vi "IC_ActiveBuffer_to_Picture.vi"(0 "ICImagingControl In":refnum<k7>, 1 "Error In (no error)":errorcluster) -> (2 "ICImagingControl Out":refnum<k7>, 3 "Picture Out":picture, 4 "SampleStartTime":dbl, 5 "Error Out":errorcluster)   [LabVIEW 2015]
uses:
  <vilib>/picture/picture.llb/Draw 8-Bit Pixmap.vi
  <vilib>/picture/picture.llb/Draw True-Color Pixmap.vi
  IC LabVIEW Extension 2.dll
  IC LabVIEW Extension 2.dll 
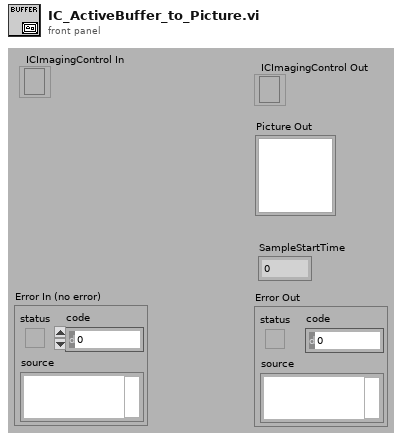
[diagram p1: front panel]
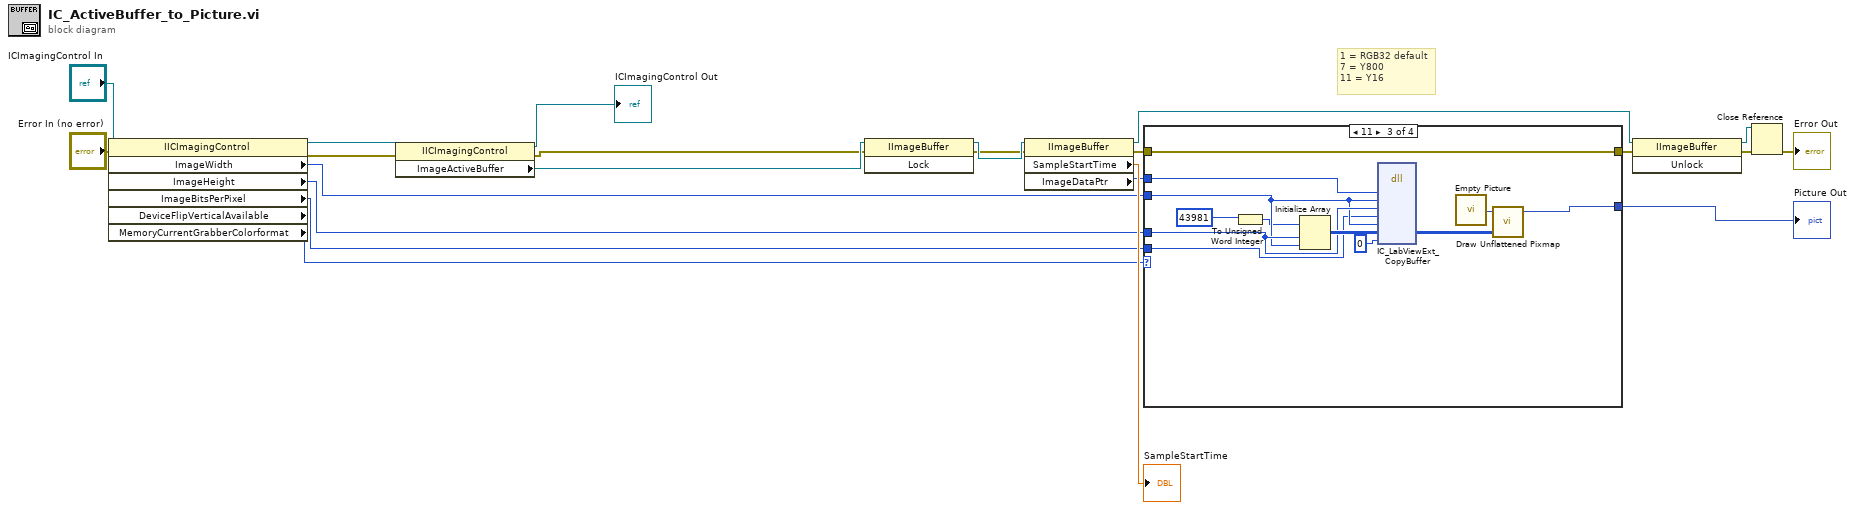
[diagram p0: block diagram]
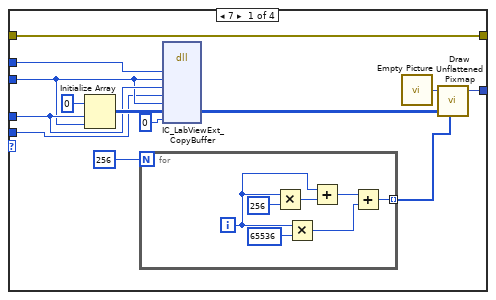
[diagram p2: hidden frame]
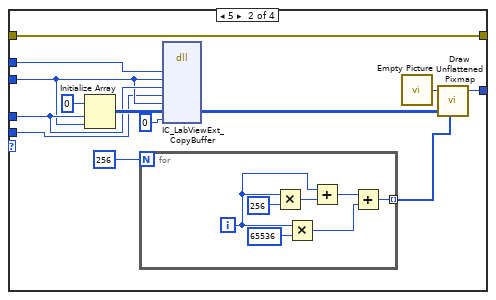
[diagram p3: hidden frame]
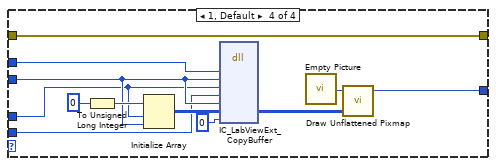
[diagram p4: hidden frame]
diagram:
  # "1 = RGB32 default\n7 = Y800\n11 = Y16"
  n1 = property class="IICImagingControl" props=["ImageWidth", "ImageHeight", "ImageBitsPerPixel", "DeviceFlipVerticalAvailable", "MemoryCurrentGrabberColorformat"](reference="ICImagingControl In", error in="Error In (no error)") -> (reference out=w6:refnum<k7>, error out=w4:errorcluster, "ImageWidth"=w12:i32, "ImageHeight"=w13:i32, "ImageBitsPerPixel"=w11:i32, "MemoryCurrentGrabberColorformat"=w14:i32)  [unwired: 1 out]
  n2 = property class="IICImagingControl"(reference=w6, error in=w4) -> (reference out=→"ICImagingControl Out":refnum<k7>, error out=w2:errorcluster, "ImageActiveBuffer"=w3:refnum<k7>)
  n3 = invoke class="IImageBuffer" method="Lock"(reference=w3, error in=w2) -> (reference out=w15:refnum<k7>, error out=w1:errorcluster)  [unwired: 1 in, 1 out]
  n4 = property class="IImageBuffer"(reference=w15, error in=w1) -> (reference out=w20:refnum<k7>, error out=w8:errorcluster, "SampleStartTime"=→"SampleStartTime":dbl, "ImageDataPtr"=w10:i32)
  n5 = case shown="11" w14 {
    tunnel: w13 -> [w28 w48 w70 w79]
    tunnel: w12 -> [w27 w47 w69 w80]
    tunnel: w11 -> [w26 w46 w68 w78]
    tunnel: w10 -> [w25 w45 w67 w77]
    tunnel: [w24 w44 w66 w76] -> w9
    tunnel: w8 -> [w23 w43 w65 w75]
    tunnel: [w23 w43 w65 w75] -> w7
    frame 7 {
      n6 = Initialize Array(u8 0, w28, w27) -> (w31:u8[][])
      n7 = for {
        N: 256 -> [_]
        tunnel: [w36] -> w32 mode=indexing
        i -> [w37]
        n8 = Multiply(x=w37, y=256) -> (x*y=w40:i32)
        n9 = Multiply(x=w37, y=65536) -> (x*y=w42:i32)
        n10 = Add(x=w37, y=w40) -> (x+y=w38:i32)
        n11 = Add(x=w38, y=w42) -> (x+y=w36:i32)
      }
      n12 = dll-call lib="IC LabVIEW Extension 2.dll " fn="IC_LabViewExt_CopyBuffer"("data"=w25, "width"=w27, "height"=w28, "bpp"=w26, "imaq_width"=w27, "imaq_ptr"=w31, "bFlip"=0) -> ("imaq_ptr"=w29:u8[][])  [unwired: 10 in, 2 out]
      n13 = call "Empty Picture"() -> ("empty picture"=w35:picture)
      n14 = call-poly <vilib>:"Draw Unflattened Pixmap.vi"("picture"=w35, "data"=w29, "color table"=w32) -> ("new picture"=w24:picture)  [unwired: 6 in]
    }
    frame 5 {
      n15 = Initialize Array(u8 0, w48, w47) -> (w51:u8[][])
      n16 = for {
        N: 256 -> [_]
        tunnel: [w56] -> w52 mode=indexing
        i -> [w57]
        n17 = Multiply(x=w57, y=256) -> (x*y=w60:i32)
        n18 = Multiply(x=w57, y=65536) -> (x*y=w62:i32)
        n19 = Add(x=w57, y=w60) -> (x+y=w58:i32)
        n20 = Add(x=w58, y=w62) -> (x+y=w56:i32)
      }
      n21 = dll-call lib="IC LabVIEW Extension 2.dll " fn="IC_LabViewExt_CopyBuffer"("data"=w45, "width"=w47, "height"=w48, "bpp"=w46, "imaq_width"=w47, "imaq_ptr"=w51, "bFlip"=0) -> ("imaq_ptr"=w49:u8[][])  [unwired: 10 in, 2 out]
      n22 = call "Empty Picture"() -> ("empty picture"=w55:picture)
      n23 = call-poly <vilib>:"Draw Unflattened Pixmap.vi"("picture"=w55, "data"=w49, "color table"=w52) -> ("new picture"=w44:picture)  [unwired: 6 in]
    }
    frame 11 {
      n24 = To Unsigned Word Integer(number=u16 43981) -> (unsigned 16bit integer=w63:u16)
      n25 = Initialize Array(w63, w70, w69) -> (w73:u16[][])
      n26 = dll-call lib="IC LabVIEW Extension 2.dll " fn="IC_LabViewExt_CopyBuffer"("data"=w67, "width"=w69, "height"=w70, "bpp"=w68, "imaq_width"=w69, "imaq_ptr"=w73, "bFlip"=0) -> ("imaq_ptr"=w71:u16[][])  [unwired: 10 in, 2 out]
      n27 = call "Empty Picture"() -> ("empty picture"=w74:picture)
      n28 = call-poly <vilib>:"Draw Unflattened Pixmap.vi"("picture"=w74, "data"=w71) -> ("new picture"=w66:picture)  [unwired: 7 in]
    }
    frame 1, Default {
      n29 = To Unsigned Long Integer(number=u8 0) -> (unsigned 32bit integer=w81:u32)
      n30 = Initialize Array(w81, w79, w80) -> (w85:u32[][])
      n31 = dll-call lib="W:/Labview/Front ends/ARPEScontrol/subvi/IC/IC LabVIEW Extension 2.dll" fn="IC_LabViewExt_CopyBuffer"("data"=w77, "width"=w80, "height"=w79, "bpp"=w78, "imaq_width"=w80, "imaq_ptr"=w85, "bFlip"=0) -> ("imaq_ptr"=w83:u32[][])  [unwired: 10 in, 2 out]
      n32 = call "Empty Picture"() -> ("empty picture"=w86:picture)
      n33 = call-poly <vilib>:"Draw Unflattened Pixmap.vi"("picture"=w86, "data (RGB format)"=w83) -> ("new picture"=w76:picture)  [unwired: 7 in]
    }
  }
  "Picture Out" <- w9
  n34 = invoke class="IImageBuffer" method="Unlock"(reference=w20, error in=w7) -> (reference out=w16:refnum<k7>, error out=w18:errorcluster)  [unwired: 1 in, 1 out]
  n35 = Close Reference(reference=w16, error in (no error)=w18) -> (error out=→"Error Out":errorcluster)
